vi "Delta_PLC_Test.vi"() -> ()   [LabVIEW 2017]
uses:
  <vilib>/NI/Modbus Library/API/Wrapper/Create TCP Master.vi
  <vilib>/NI/Modbus Library/API/master/Modbus Master.lvclass
  <vilib>/NI/Modbus Library/API/Wrapper/API Main.lvlib
panel:
  in  "number of register":u16=2
  in  "starting address":u16=60021
  in  "address":string="192.168.1.5"
  in  "error in":errorcluster
  in  "stop":bool
  out "register values":u16[](array[numeric])
  out "error out":errorcluster
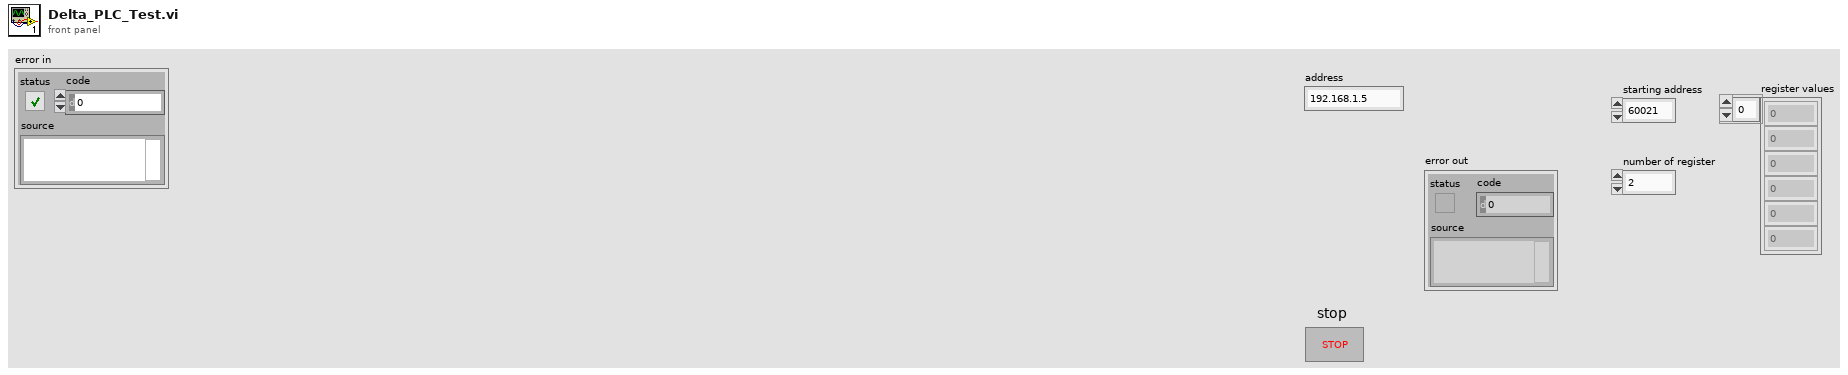
[diagram p1: front panel]
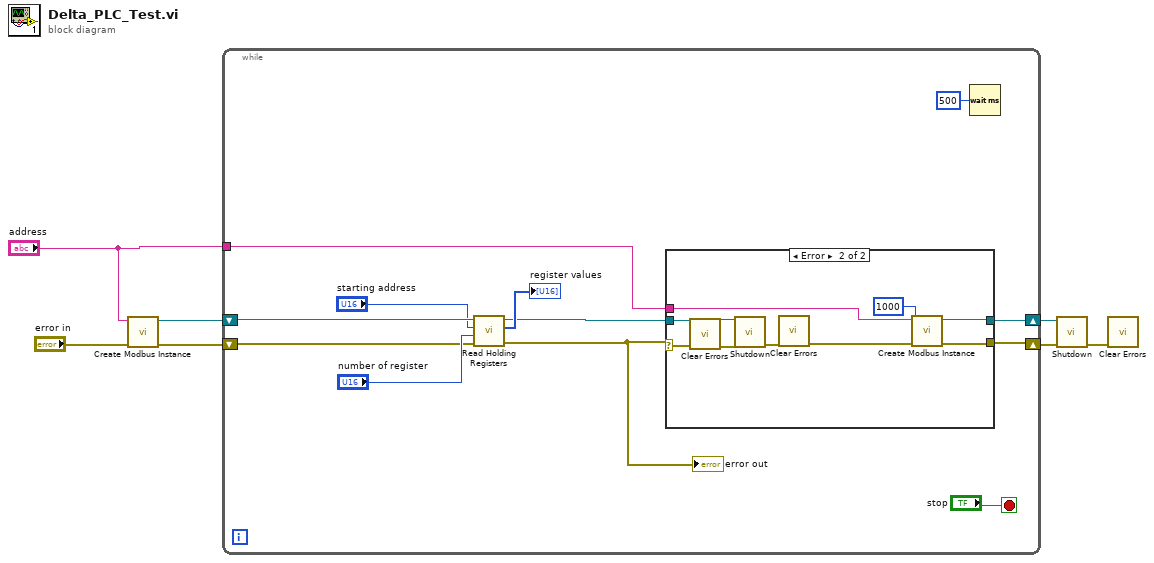
[diagram p0: block diagram]
diagram:
  n1 = call-poly <vilib>:"Create Modbus Instance.vi"("error in"="error in", "address"="address") -> ("error out"=w5:errorcluster, "TCP master instance"=w4:refnum<class "Modbus Master.lvclass">)  [unwired: 8 in]
  n2 = while {
    shift-right: [w19] -> w7
    shift-left: w4 -> [w15]
    shift-right: [w18] -> w6
    shift-left: w5 -> [w16]
    tunnel: "address" -> [w10]
    stop <- "stop" stop-if-true
    n3 = call-dynamic "Read Holding Registers.vi"("error in"=w16, "number of inputs"="number of register", "starting address"="starting address", "Modbus master in"=w15) -> ("error out"=w12:errorcluster, "register values"=→"register values":u16[], "Modbus master out"=w11:refnum<class "Modbus Master.lvclass">)  [unwired: 5 in]
    "error out" <- w12
    n4 = case shown="Error" w12 {
      selector: w12 -> [w20 w30]
      tunnel: w11 -> [w21 w28]
      tunnel: [w21 w25] -> w19
      tunnel: [w20 w24] -> w18
      tunnel: w10 -> [_ w22]
      frame No Error {
      }
      frame Error {
        n5 = call <vilib>:"Clear Errors.vi"("error in (no error)"=w30) -> ("error out"=w29:errorcluster)  [unwired: 5 in, 1 out]
        n6 = call-dynamic "Shutdown.vi"("error in"=w29, "Modbus master in"=w28) -> ("error out"=w27:errorcluster)  [unwired: 9 in]
        n7 = call <vilib>:"Clear Errors.vi"("error in (no error)"=w27) -> ("error out"=w26:errorcluster)  [unwired: 5 in, 1 out]
        n8 = call-poly <vilib>:"Create Modbus Instance.vi"("error in"=w26, "connect timeout ms"=1000, "address"=w22) -> ("error out"=w24:errorcluster, "TCP master instance"=w25:refnum<class "Modbus Master.lvclass">)  [unwired: 7 in]
      }
    }
    n9 = Wait (ms)(milliseconds to wait=u32 500) -> ()  [unwired: 1 out]
  }
  n10 = call-dynamic "Shutdown.vi"("error in"=w6, "Modbus master in"=w7) -> ("error out"=w2:errorcluster)  [unwired: 9 in]
  n11 = call <vilib>:"Clear Errors.vi"("error in (no error)"=w2) -> ()  [unwired: 5 in, 2 out]
